vi "VISJS Viewer.vi"(4 "Extra Scripts":string, 5 "FileDependency out":map{path, T1}(c390), 6 "Options":string, 7 "OpenWebBrowser(False)":bool, 8 "error in":errorcluster, 9 "Embedd VISJS Librarya in HTMl File(False)":bool, 10 "HTMLFilePath":path, 11 "LibraryDependency":map{path, T3}(c390)) -> (0 "error out":errorcluster, 3 "HTMLFileContent":string)   [LabVIEW 2020, in "VISJS Viewer.lvlib"] (continued)
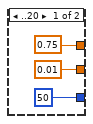
[diagram p2: hidden frame]
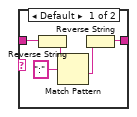
[diagram p6: hidden frame]
d=r[2];e<s&&(e=s,C=n,I=a,i=d)}}return[C,e,I,i]}},{key:\"_getEnergy\",value:function(g){var t=lh(this.E_sums[g],2),A=t[0],e=t[1];return[Math.sqrt(Math.pow(A,2)+Math.pow(e,2)),A,e]}},{key:\"_moveNode\",value:function(g,t,A){for(var e=this.body.nodeIndices,C=this.body.nodes,I=0,i=0,o=0,n=C[g].x,r=C[g].y,s=this.K_matrix[g],a=this.L_matrix[g],d=0;d<e.length;d++){var h=e[d];if(h!==g){var l=C[h].x,c=C[h].y,u=s[h],p=a[h],f=1/Math.pow(Math.pow(n-l,2)+Math.pow(r-c,2),1.5);I+=u*(1-p*Math.pow(r-c,2)*f),i+=u*(p*(n-l)*(r-c)*f),o+=u*(1-p*Math.pow(n-l,2)*f)}}var v=(t/I+A/i)/(i/I-o/i),y=-(i*v+t)/I;C[g].x+=y,C[g].y+=v,this._updateE_matrix(g)}},{key:\"_createL_matrix\",value:function(g){var t=this.body.nodeIndices,A=this.springLength;this.L_matrix=[];for(var e=0;e<t.length;e++){this.L_matrix[t[e]]={};for(var C=0;C<t.length;C++)this.L_matrix[t[e]][t[C]]=A*g[t[e]][t[C]]}}},{key:\"_createK_matrix\",value:function(g){var t=this.body.nodeIndices,A=this.springConstant;this.K_matrix=[];for(var e=0;e<t.length;e++){this.K_matrix[t[e]]={};for(var C=0;C<t.length;C++)this.K_matrix[t[e]][t[C]]=A*Math.pow(g[t[e]][t[C]],-2)}}},{key:\"_createE_matrix\",value:function(){var g=this.body.nodeIndices,t=this.body.nodes;this.E_matrix={},this.E_sums={};for(var A=0;A<g.length;A++)this.E_matrix[g[A]]=[];for(var e=0;e<g.length;e++){for(var C=g[e],I=t[C].x,i=t[C].y,o=0,n=0,r=e;r<g.length;r++){var s=g[r];if(s!==C){var a=t[s].x,d=t[s].y,h=1/Math.sqrt(Math.pow(I-a,2)+Math.pow(i-d,2));this.E_matrix[C][r]=[this.K_matrix[C][s]*(I-a-this.L_matrix[C][s]*(I-a)*h),this.K_matrix[C][s]*(i-d-this.L_matrix[C][s]*(i-d)*h)],this.E_matrix[s][e]=this.E_matrix[C][r],o+=this.E_matrix[C][r][0],n+=this.E_matrix[C][r][1]}}this.E_sums[C]=[o,n]}}},{key:\"_updateE_matrix\",value:function(g){for(var t=this.body.nodeIndices,A=this.body.nodes,e=this.E_matrix[g],C=this.K_matrix[g],I=this.L_matrix[g],i=A[g].x,o=A[g].y,n=0,r=0,s=0;s<t.length;s++){var a=t[s];if(a!==g){var d=e[s],h=d[0],l=d[1],c=A[a].x,u=A[a].y,p=1/Math.sqrt(Math.pow(i-c,2)+Math.pow(o-u,2)),f=C[a]*(i-c-I[a]*(i-c)*p),v=C[a]*(o-u-I[a]*(o-u)*p);e[s]=[f,v],n+=f,r+=v;var y=this.E_sums[a];y[0]+=f-h,y[1]+=v-l}}this.E_sums[g]=[n,r]}}]),g}();function gB(g,t,A){var e,C,I,i,o=this;if(!(this instanceof gB))throw new SyntaxError(\"Constructor must be called with the new operator\");this.options={},this.defaultOptions={locale:\"en\",locales:ny,clickToUse:!1},fe(this.options,this.defaultOptions),this.body={container:g,nodes:{},nodeIndices:[],edges:{},edgeIndices:[],emitter:{on:je(e=this.on).call(e,this),off:je(C=this.off).call(C,this),emit:je(I=this.emit).call(I,this),once:je(i=this.once).call(i,this)},eventListeners:{onTap:function(){},onTouch:function(){},onDoubleTap:function(){},onHold:function(){},onDragStart:function(){},onDrag:function(){},onDragEnd:function(){},onMouseWheel:function(){},onPinch:function(){},onMouseMove:function(){},onRelease:function(){},onContext:function(){}},data:{nodes:null,edges:null},functions:{createNode:function(){},createEdge:function(){},getPointer:function(){}},modules:{},view:{scale:1,translation:{x:0,y:0}},selectionBox:{show:!1,position:{start:{x:0,y:0},end:{x:0,y:0}}}},this.bindEventListeners(),this.images=new sy((function(){return o.body.emitter.emit(\"_requestRedraw\")})),this.groups=new Gm,this.canvas=new CP(this.body),this.selectionHandler=new yM(this.body,this.canvas),this.interactionHandler=new sP(this.body,this.canvas,this.selectionHandler),this.view=new IP(this.body,this.canvas),this.renderer=new gP(this.body,this.canvas),this.physics=new HR(this.body),this.layoutEngine=new ZM(this.body),this.clustering=new $R(this.body),this.manipulation=new jM(this.body,this.canvas,this.selectionHandler,this.interactionHandler),this.nodesHandler=new YN(this.body,this.images,this.groups,this.layoutEngine),this.edgesHandler=new FR(this.body,this.images,this.groups),this.body.modules.kamadaKawai=new $M(this.body,150,.05),this.body.modules.clustering=this.clustering,this.canvas._create(),this.setOptions(A),this.setData(t)}He(gB.prototype),gB.prototype.setOptions=function(g){var t=this;if(null===g&&(g=void 0),void 0!==g){!0===Dv.validate(g,KM)&&console.error(\"%cErrors have been found in the supplied options object.\",Tv);if(Xf([\"locale\",\"locales\",\"clickToUse\"],this.options,g),void 0!==g.locale&&(g.locale=function(g,t){try{var A=lh(t.split(/[-_ /]/,2),2),e=A[0],C=A[1],I=null!=e?e.toLowerCase():null,i=null!=C?C.toUpperCase():null;if(I&&i){var o,n=I+\"-\"+i;if(Object.prototype.hasOwnProperty.call(g,n))return n;console.warn(bh(o=\"Unknown variant \".concat(i,\" of language \")).call(o,I,\".\"))}if(I){var r=I;if(Object.prototype.hasOwnProperty.call(g,r))return r;console.warn(\"Unknown language \".concat(I))}return console.warn(\"Unknown locale \".concat(t,\", falling back to English.\")),\"en\"}catch(g){return console.error(g),console.warn(\"Unexpected error while normalizing locale \".concat(t,\", falling back to English.\")),\"en\"}}(g.locales||this.options.locales,g.locale)),g=this.layoutEngine.setOptions(g.layout,g),this.canvas.setOptions(g),this.groups.setOptions(g.groups),this.nodesHandler.setOptions(g.nodes),this.edgesHandler.setOptions(g.edges),this.physics.setOptions(g.physics),this.manipulation.setOptions(g.manipulation,g,this.options),this.interactionHandler.setOptions(g.interaction),this.renderer.setOptions(g.interaction),this.selectionHandler.setOptions(g.interaction),void 0!==g.groups&&this.body.emitter.emit(\"refreshNodes\"),\"configure\"in g&&(this.configurator||(this.configurator=new xv(this,this.body.container,HM,this.canvas.pixelRatio,XM)),this.configurator.setOptions(g.configure)),this.configurator&&!0===this.configurator.options.enabled){var A={nodes:{},edges:{},layout:{},interaction:{},manipulation:{},physics:{},global:{}};qf(A.nodes,this.nodesHandler.options),qf(A.edges,this.edgesHandler.options),qf(A.layout,this.layoutEngine.options),qf(A.interaction,this.selectionHandler.options),qf(A.interaction,this.renderer.options),qf(A.interaction,this.interactionHandler.options),qf(A.manipulation,this.manipulation.options),qf(A.physics,this.physics.options),qf(A.global,this.canvas.options),qf(A.global,this.options),this.configurator.setModuleOptions(A)}void 0!==g.clickToUse?!0===g.clickToUse?void 0===this.activator&&(this.activator=new kv(this.canvas.frame),this.activator.on(\"change\",(function(){t.body.emitter.emit(\"activate\")}))):(void 0!==this.activator&&(this.activator.destroy(),delete this.activator),this.body.emitter.emit(\"activate\")):this.body.emitter.emit(\"activate\"),this.canvas.setSize(),this.body.emitter.emit(\"startSimulation\")}},gB.prototype._updateVisibleIndices=function(){var g=this.body.nodes,t=this.body.edges;for(var A in this.body.nodeIndices=[],this.body.edgeIndices=[],g)Object.prototype.hasOwnProperty.call(g,A)&&(this.clustering._isClusteredNode(A)||!1!==g[A].options.hidden||this.body.nodeIndices.push(g[A].id));for(var e in t)if(Object.prototype.hasOwnProperty.call(t,e)){var C=t[e],I=g[C.fromId],i=g[C.toId],o=void 0!==I&&void 0!==i;!this.clustering._isClusteredEdge(e)&&!1===C.options.hidden&&o&&!1===I.options.hidden&&!1===i.options.hidden&&this.body.edgeIndices.push(C.id)}},gB.prototype.bindEventListeners=function(){var g=this;this.body.emitter.on(\"_dataChanged\",(function(){g.edgesHandler._updateState(),g.body.emitter.emit(\"_dataUpdated\")})),this.body.emitter.on(\"_dataUpdated\",(function(){g.clustering._updateState(),g._updateVisibleIndices(),g._updateValueRange(g.body.nodes),g._updateValueRange(g.body.edges),g.body.emitter.emit(\"startSimulation\"),g.body.emitter.emit(\"_requestRedraw\")}))},gB.prototype.setData=function(g){if(this.body.emitter.emit(\"resetPhysics\"),this.body.emitter.emit(\"_resetData\"),this.selectionHandler.unselectAll(),g&&g.dot&&(g.nodes||g.edges))throw new SyntaxError('Data must contain either parameter \"dot\" or  parameter pair \"nodes\" and \"edges\", but not both.');if(this.setOptions(g&&g.options),g&&g.dot){console.warn(\"The dot property has been deprecated. Please use the static convertDot method to convert DOT into vis.network format and use the normal data format with nodes and edges. This converter is used like this: var data = vis.network.convertDot(dotString);\");var t=Cy(g.dot);this.setData(t)}else if(g&&g.gephi){console.warn(\"The gephi property has been deprecated. Please use the static convertGephi method to convert gephi into vis.network format and use the normal data format with nodes and edges. This converter is used like this: var data = vis.network.convertGephi(gephiJson);\");var A=iy(g.gephi);this.setData(A)}else this.nodesHandler.setData(g&&g.nodes,!0),this.edgesHandler.setData(g&&g.edges,!0),this.body.emitter.emit(\"_dataChanged\"),this.body.emitter.emit(\"_dataLoaded\"),this.body.emitter.emit(\"initPhysics\")},gB.prototype.destroy=function(){for(var g in this.body.emitter.emit(\"destroy\"),this.body.emitter.off(),this.off(),delete this.groups,delete this.canvas,delete this.selectionHandler,delete this.interactionHandler,delete this.view,delete this.renderer,delete this.physics,delete this.layoutEngine,delete this.clustering,delete this.manipulation,delete this.nodesHandler,delete this.edgesHandler,delete this.configurator,delete this.images,this.body.nodes)Object.prototype.hasOwnProperty.call(this.body.nodes,g)&&delete this.body.nodes[g];for(var t in this.body.edges)Object.prototype.hasOwnProperty.call(this.body.edges,t)&&delete this.body.edges[t];Qf(this.body.container)},gB.prototype._updateValueRange=function(g){var t,A=void 0,e=void 0,C=0;for(t in g)if(Object.prototype.hasOwnProperty.call(g,t)){var I=g[t].getValue();void 0!==I&&(A=void 0===A?I:Math.min(I,A),e=void 0===e?I:Math.max(I,e),C+=I)}if(void 0!==A&&void 0!==e)for(t in g)Object.prototype.hasOwnProperty.call(g,t)&&g[t].setValueRange(A,e,C)},gB.prototype.isActive=function(){return!this.activator||this.activator.active},gB.prototype.setSize=function(){return this.canvas.setSize.apply(this.canvas,arguments)},gB.prototype.canvasToDOM=function(){return this.canvas.canvasToDOM.apply(this.canvas,arguments)},gB.prototype.DOMtoCanvas=function(){return this.canvas.DOMtoCanvas.apply(this.canvas,arguments)},gB.prototype.findNode=function(){return this.clustering.findNode.apply(this.clustering,arguments)},gB.prototype.isCluster=function(){return this.clustering.isCluster.apply(this.clustering,arguments)},gB.prototype.openCluster=function(){return this.clustering.openCluster.apply(this.clustering,arguments)},gB.prototype.cluster=function(){return this.clustering.cluster.apply(this.clustering,arguments)},gB.prototype.getNodesInCluster=function(){return this.clustering.getNodesInCluster.apply(this.clustering,arguments)},gB.prototype.clusterByConnection=function(){return this.clustering.clusterByConnection.apply(this.clustering,arguments)},gB.prototype.clusterByHubsize=function(){return this.clustering.clusterByHubsize.apply(this.clustering,arguments)},gB.prototype.updateClusteredNode=function(){return this.clustering.updateClusteredNode.apply(this.clustering,arguments)},gB.prototype.getClusteredEdges=function(){return this.clustering.getClusteredEdges.apply(this.clustering,arguments)},gB.prototype.getBaseEdge=function(){return this.clustering.getBaseEdge.apply(this.clustering,arguments)},gB.prototype.getBaseEdges=function(){return this.clustering.getBaseEdges.apply(this.clustering,arguments)},gB.prototype.updateEdge=function(){return this.clustering.updateEdge.apply(this.clustering,arguments)},gB.prototype.clusterOutliers=function(){return this.clustering.clusterOutliers.apply(this.clustering,arguments)},gB.prototype.getSeed=function(){return this.layoutEngine.getSeed.apply(this.layoutEngine,arguments)},gB.prototype.enableEditMode=function(){return this.manipulation.enableEditMode.apply(this.manipulation,arguments)},gB.prototype.disableEditMode=function(){return this.manipulation.disableEditMode.apply(this.manipulation,arguments)},gB.prototype.addNodeMode=function(){return this.manipulation.addNodeMode.apply(this.manipulation,arguments)},gB.prototype.editNode=function(){return this.manipulation.editNode.apply(this.manipulation,arguments)},gB.prototype.editNodeMode=function(){return console.warn(\"Deprecated: Please use editNode instead of editNodeMode.\"),this.manipulation.editNode.apply(this.manipulation,arguments)},gB.prototype.addEdgeMode=function(){return this.manipulation.addEdgeMode.apply(this.manipulation,arguments)},gB.prototype.editEdgeMode=function(){return this.manipulation.editEdgeMode.apply(this.manipulation,arguments)},gB.prototype.deleteSelected=function(){return this.manipulation.deleteSelected.apply(this.manipulation,arguments)},gB.prototype.getPositions=function(){return this.nodesHandler.getPositions.apply(this.nodesHandler,arguments)},gB.prototype.getPosition=function(){return this.nodesHandler.getPosition.apply(this.nodesHandler,arguments)},gB.prototype.storePositions=function(){return this.nodesHandler.storePositions.apply(this.nodesHandler,arguments)},gB.prototype.moveNode=function(){return this.nodesHandler.moveNode.apply(this.nodesHandler,arguments)},gB.prototype.getBoundingBox=function(){return this.nodesHandler.getBoundingBox.apply(this.nodesHandler,arguments)},gB.prototype.getConnectedNodes=function(g){return void 0!==this.body.nodes[g]?this.nodesHandler.getConnectedNodes.apply(this.nodesHandler,arguments):this.edgesHandler.getConnectedNodes.apply(this.edgesHandler,arguments)},gB.prototype.getConnectedEdges=function(){return this.nodesHandler.getConnectedEdges.apply(this.nodesHandler,arguments)},gB.prototype.startSimulation=function(){return this.physics.startSimulation.apply(this.physics,arguments)},gB.prototype.stopSimulation=function(){return this.physics.stopSimulation.apply(this.physics,arguments)},gB.prototype.stabilize=function(){return this.physics.stabilize.apply(this.physics,arguments)},gB.prototype.getSelection=function(){return this.selectionHandler.getSelection.apply(this.selectionHandler,arguments)},gB.prototype.setSelection=function(){return this.selectionHandler.setSelection.apply(this.selectionHandler,arguments)},gB.prototype.getSelectedNodes=function(){return this.selectionHandler.getSelectedNodeIds.apply(this.selectionHandler,arguments)},gB.prototype.getSelectedEdges=function(){return this.selectionHandler.getSelectedEdgeIds.apply(this.selectionHandler,arguments)},gB.prototype.getNodeAt=function(){var g=this.selectionHandler.getNodeAt.apply(this.selectionHandler,arguments);return void 0!==g&&void 0!==g.id?g.id:g},gB.prototype.getEdgeAt=function(){var g=this.selectionHandler.getEdgeAt.apply(this.selectionHandler,arguments);return void 0!==g&&void 0!==g.id?g.id:g},gB.prototype.selectNodes=function(){return this.selectionHandler.selectNodes.apply(this.selectionHandler,arguments)},gB.prototype.selectEdges=function(){return this.selectionHandler.selectEdges.apply(this.selectionHandler,arguments)},gB.prototype.unselectAll=function(){this.selectionHandler.unselectAll.apply(this.selectionHandler,arguments),this.selectionHandler.commitWithoutEmitting.apply(this.selectionHandler),this.redraw()},gB.prototype.redraw=function(){return this.renderer.redraw.apply(this.renderer,arguments)},gB.prototype.getScale=function(){return this.view.getScale.apply(this.view,arguments)},gB.prototype.getViewPosition=function(){return this.view.getViewPosition.apply(this.view,arguments)},gB.prototype.fit=function(){return this.view.fit.apply(this.view,arguments)},gB.prototype.moveTo=function(){return this.view.moveTo.apply(this.view,arguments)},gB.prototype.focus=function(){return this.view.focus.apply(this.view,arguments)},gB.prototype.releaseNode=function(){return this.view.releaseNode.apply(this.view,arguments)},gB.prototype.getOptionsFromConfigurator=function(){var g={};return this.configurator&&(g=this.configurator.getOptions.apply(this.configurator)),g};var tB=Cy;g.DataSet=mD,g.DataView=bD,g.Network=gB,g.NetworkImages=sy,g.Queue=fD,g.data=xD,g.networkDOTParser=Iy,g.networkGephiParser=oy,g.networkOptions=JM,g.parseDOTNetwork=tB,g.parseGephiNetwork=iy}));\n//# sourceMappingURL=vis-network.min.js.map\n"  # https://visjs.github.io/vis-network/standalone/umd/vis-network.min.js 2024-08-26T06:20:20.413Z
  n1 = Array Size(array=w28) -> (size(s)=w29:i32)
  n2 = for {
    tunnel: "LibraryDependency" -> [w50] mode=indexing
    tunnel: "{from: \"%s\",to: \"%s\",arrows: \"to\",id: \"E%d\"}\n" -> [w47]
    tunnel: [w46] -> w25 mode=concatenating
    shift-right: [w44] -> _
    shift-left: 0 -> [w45]
    tunnel: "FileDependency out" -> [w43]
    tunnel: [w42] -> w4 mode=concatenating
    tunnel: [w41] -> _ mode=indexing
    i -> [w41]
    n3 = Unbundle By Name(w50) -> ("Path"=w49:path, "LibraryDependentInfo.DependentLibrary"=w48:map{path, set{path}})
    n4 = for {
      tunnel: w49 -> [w68]
      tunnel: w48 -> [w65] mode=indexing
      tunnel: w47 -> [w67]
      tunnel: [w66] -> w46 mode=indexing
      shift-right: [w57] -> w44
      shift-left: w45 -> [w61]
      tunnel: w43 -> [w60]
      tunnel: [w55] -> w42 mode=indexing
      n5 = Unbundle By Name(w65) -> ("Path"=w64:path, "Callers"=w59:set{path})
      n6 = for {
        tunnel: w60 -> [w93]
        tunnel: w59 -> [w92] mode=indexing
        shift-right: [w88] -> w53
        shift-left: map{string, set{string}} {} ("Size: 0") -> [w90]
        n7 = Look In Map(map=w93, key=w92) -> (value=w91:T1)  [unwired: 1 in, 1 out]
        n8 = Unbundle By Name(w91) -> ("FullQualifierName"=w85:string, "Path"=w87:path)
        n9 = call <vilib>:"Get File Extension.vi"("file"=w87) -> ("lowercase file extension"=w86:string)  [unwired: 6 in, 4 out]
        n10 = case shown="\"lvclass\"" w86 {
          tunnel: w85 -> [w98 w99]
          tunnel: [w94 w99] -> w84
          frame Default {
            n11 = Reverse String(1:w98) -> (0:w97:string)
            n12 = Match Pattern(string=w97, regular expression=":") -> (after substring=w95:string)  [unwired: 1 in, 3 out]
            n13 = Reverse String(1:w95) -> (0:w94:string)
          }
          frame "lvclass" {
          }
        }
        n14 = Strip Path(path=w87) -> (name=w89:string)  [unwired: 1 out]
        n15 = in-place {
          in-place-border: w89 -> [w102]
          n16 = in-place-map #1(w90, w84) -> (w103:set{string})  [unwired: 1 in, 1 out]
          n17 = Insert Into Set(10:w102, 11:w103) -> (3:w101:set{string})  [unwired: 1 out]
          n18 = in-place-map #1(w101, LVMapReplaceAction."Add or Modify Entry" ("action")) -> (w88:map{string, set{string}})  [unwired: 2 out]
        }
      }
      n19 = Increment(x=w61) -> (x+1=w57:i32)
      n20 = for {
        tunnel: w53 -> [w75] mode=indexing
        tunnel: [w72] -> w52 mode=indexing
        n21 = Unbundle(w75) -> ("FullQualifierName"=w70:string, w74:set{string})
        n22 = for {
          tunnel: w74 -> [w83] mode=indexing
          tunnel: [w83] -> w73 mode=indexing if=w81
          tunnel: w70 -> [w82]
          n23 = Not Equal?(x=w82, y=w83) -> (x != y?=w81:bool)
        }
        n24 = call <vilib>:"Join Strings.vi"("Separator (,)"=", ", "Strings In"=w73) -> ("String"=w71:string)  [unwired: 1 in]
        n25 = case shown="Default" w70 {
          selector: w70 -> [_ w80]
          tunnel: w71 -> [w76 w78]
          tunnel: [w76 w77] -> w72
          frame "" {
          }
          frame Default {
            n26 = Format Into String(format string="%s  [%s]", w80, w78) -> (resulting string=w77:string)  [unwired: 2 in, 1 out]
          }
        }
      }
      n27 = call "VISJS Viewer_EscapePath.vi"("Path"=w68) -> ("File Path"=w63:string)  [unwired: 10 in]
      n28 = call "VISJS Viewer_EscapePath.vi"("Path"=w64) -> ("File Path"=w62:string)  [unwired: 10 in]
      n29 = call <vilib>:"Join Strings.vi"("Separator (,)"="<BR> ", "Strings In"=w52) -> ("String"=w56:string)  [unwired: 1 in]
      n30 = Format Into String(format string="E%d : \"%s\"\n", w57, w56) -> (resulting string=w55:string)  [unwired: 2 in, 1 out]
      n31 = Format Into String(format string=w67, w63, w62, w57) -> (resulting string=w66:string)  [unwired: 2 in, 1 out]
    }
  }
  n32 = for {
    tunnel: "LibraryDependency" -> [w122] mode=indexing
    tunnel: "{id: \"%s\",size: 150,label:\"%s\",color: \"#%02X%02X%02x\",cid: \"%s\",shape: \"box\"}\n" -> [w121]
    tunnel: w29 -> [w119]
    tunnel: w28 -> [w117]
    tunnel: [w111] -> w27 mode=indexing
    i -> [w120]
    w105 = ":" ("search string")
    n33 = Unbundle By Name(w122) -> ("Path"=w116:path, "LibraryDependentInfo.FullQualifierName"=w106:string)
    n34 = Quotient & Remainder(x=w120, y=w119) -> (x-y*floor(x/y)=w118:i32)  [unwired: 1 out]
    n35 = Index Array(array=w117, index=w118) -> (element=w115:u32)
    n36 = call <vilib>:"Color to RGB.vi"("Color"=w115) -> ("R"=w114:u8, "G"=w113:u8, "B"=w112:u8)  [unwired: 1 out]
    n37 = Match Pattern(string=w106, regular expression=w105) -> (before substring=w104:string)  [unwired: 1 in, 3 out]
    n38 = Search and Replace String(replace all?=TRUE ("replace all? (F)"), input string=w106, search string=w105, replace string="\\n" ("replace string (\"\")")) -> (result string=w108:string)  [unwired: 4 in, 3 out]
    n39 = call "VISJS Viewer_EscapePath.vi"("Path"=w116) -> ("File Path"=w110:string)  [unwired: 10 in]
    n40 = Format Into String(format string=w121, w110, w108, w114, w113, w112, w104) -> (resulting string=w111:string)  [unwired: 2 in, 1 out]
  }
  n41 = Empty String/Path?(string/path="HTMLFilePath") -> (empty?=w36:bool)
  n42 = Compound Arithmetic op=AND(w36, "OpenWebBrowser(False)") -> (w35:bool)
  n43 = Collection Size(1:"LibraryDependency") -> (0:w11:i32)
  n44 = case shown="21.." w11 {
    tunnel: [0.75 0.75] -> w8
    tunnel: [0.01 0.01] -> w7
    tunnel: [50 125] -> w6
    frame ..20 {
    }
    frame 21.. {
    }
  }
  n45 = case shown="True" w35 {
    tunnel: "HTMLFilePath" -> [w129 _]
    tunnel: [w129 w130] -> w18
    frame False {
    }
    frame True {
      n46 = Temporary Directory() -> (w132:path)
      n47 = Build Path(base path=w132, name or relative path=path "VISJS_Viewer.html") -> (appended path=w130:path)
    }
  }
  n48 = Format Into String(format string=w9, w8, w7, w6) -> (resulting string=w10:string)  [unwired: 2 in, 1 out]
  n49 = call <vilib>:"Join Strings.vi"("Strings In"=w27) -> ("String"=w26:string)  [unwired: 2 in]
  n50 = Select(t=w39, s="Embedd VISJS Librarya in HTMl File(False)", f="<script src=\"https://visjs.github.io/vis-network/standalone/umd/vis-network.min.js\"></script>") -> (s? t:f=w32:string)
  n51 = Empty String/Path?(string/path="Options") -> (empty?=w15:bool)
  n52 = Select(t=w10, s=w15, f="Options") -> (s? t:f=w13:string)
  n53 = call <vilib>:"Join Strings.vi"("Strings In"=w25) -> ("String"=w24:string)  [unwired: 2 in]
  n54 = call <vilib>:"Join Strings.vi"("Strings In"=w4) -> ("String"=w3:string)  [unwired: 2 in]
  n55 = Build Array(w32, w13, w26, w24, "Extra Scripts", w3) -> (w31:string[])
  n56 = for {
    shift-right: [w135] -> w17
    shift-left: "\n<html lang=\"en\">\n  <head>\n    <title>Vis Network | Example Applications | Disassembler</title>\n    <style type=\"text/css\">\n      #mynetwork {\n        width: 100%;\n        height: 80vh; /* Adjust height so the information appears at the bottom */\n        border: 0px solid lightgray;\n      }\n      #edgeInfo {\n        padding: 10px;\n        background-color: #f9f9f9;\n        border-top: 1px solid #ddd;\n      }\n    </style>\n    <<VISJS>>\n  </head>\n  <body>\n    <div id=\"mynetwork\"></div>\n    <div id=\"edgeInfo\">Click on an edge to see the dependency information here.</div>\n    <script type=\"text/javascript\">\n\nconst options = {\n<<OPTIONS>>\n};\n\nvar nodes = new vis.DataSet([\n<<NODES>>\n]);\n\n\nvar edges = new vis.DataSet([\n<<EDGES>>\n]);\n\nconst edgeInfoMap = {\n <<EDGEDEPENDECY>>\n};\n\n\n      var container = document.getElementById(\"mynetwork\");\n      var data = { nodes: nodes, edges: edges };\n      var gph = new vis.Network(container, data, options);\n/*\ngph.fit({\n animation: false, // Smooth transition\n minZoomLevel: .1, // Prevent zooming out too far\n maxZoomLevel: 10  // Allow zooming in more\n});\n*/\n   gph.on(\"click\", function (params) {\n  const edgeInfoElement = document.getElementById(\"edgeInfo\");\n  \n  // Check if a node is clicked\n  const nodeId = this.getNodeAt(params.pointer.DOM);\n  if (nodeId) {\n    // Get all edges where the nodeId is the \"from\" node\n    const connectedEdges = edges.get({\n      filter: (edge) => edge.from === nodeId,\n    });\n\nif (connectedEdges.length > 0) {\n  let allEdgeInfo = \"\";\n  connectedEdges.forEach((edge, index) => {\n    const edgeInfo = edgeInfoMap[edge.id] || \"No info available for this edge.\";\n    const bgColor = index % 2 === 0 ? \"#f0f0f0\" : \"#ffffff\"; // Alternate background color\n    allEdgeInfo += `<div style=\"background-color: ${bgColor}; padding: 5px;\">${edgeInfo}</div>`;\n  });\n  edgeInfoElement.innerHTML = allEdgeInfo;\n} else {\n      edgeInfoElement.innerHTML = \"No outgoing edges from this node.\";\n    }\n    return;\n  }\n\n  // Check if an edge is clicked\n  const edgeId = this.getEdgeAt(params.pointer.DOM);\n  if (edgeId) {\n    edgeInfoElement.innerHTML = edgeInfoMap[edgeId] || \"No info available for this edge.\";\n    return;\n  }\n\n  // Default message if neither node nor edge is clicked\n  edgeInfoElement.innerHTML = \"Click on an edge or node to see the dependency information here.\";\n});\n\n\n<<EXTRASCRIPTS>>\n    </script>\n  </body>\n</html>\n" -> [w136]
    tunnel: string[] [" <<VISJS>>", "<<OPTIONS>>", "<<NODES>>", "<<EDGES>>", "<<EXTRASCRIPTS>>", " <<EDGEDEPENDECY>>"] -> [w134] mode=indexing
    tunnel: w31 -> [w133] mode=indexing
    n57 = Search and Replace String(input string=w136, search string=w134, replace string=w133) -> (result string=w135:string)  [unwired: 5 in, 3 out]
  }
  "HTMLFileContent" <- w17
  n58 = Empty String/Path?(string/path=w18) -> (empty?=w23:bool)
  n59 = case shown="False" w23 {
    tunnel: w18 -> [w140 _]
    tunnel: "error in" -> [w139 w141]
    tunnel: [w138 w141] -> w21
    tunnel: w17 -> [w137 _]
    frame False {
      n60 = Write to Text File(file (use dialog)=w140, text=w137, error in=w139) -> (error out=w138:errorcluster)  [unwired: 1 in, 2 out]
    }
    frame True {
    }
  }
  n61 = case shown="True" "OpenWebBrowser(False)" {
    tunnel: w21 -> [w142 w145]
    tunnel: [w142 w144] -> w20
    tunnel: w18 -> [_ w143]
    frame False {
    }
    frame True {
      n62 = call-poly <vilib>:"Open URL in Default Browser.vi"("error in (no error)"=w145, "path"=w143) -> ("error out"=w144:errorcluster)  [unwired: 4 in, 1 out]
    }
  }
  "error out" <- w20
